vi "Desktop Main.vi"() -> ()   [LabVIEW 2016]
doc: "This VI implements the framework and scheduler for your robotics program. It should not be necessary to modify the framework. You are expected to add your code to the VIs called from Robot Main - the ones located in the Team Code folder within the project."
uses:
  Vision Server/Vision Server.lvclass
panel:
  in  "ADB Path":path caption="ADB path (if not in Windows PATH)"
  out "Distance":dbl
  in  "Goal Height":dbl
  out "Angle":dbl
  out "Connected?":bool
  out "Targets Detected:":i32
  out "Coords":cluster{"X":dbl, "Y":dbl}[](graph) caption="Frist Target Coordinates"
  out "Time Delay":u32(graph)
  in  "stop":bool
  in  "error in":errorcluster
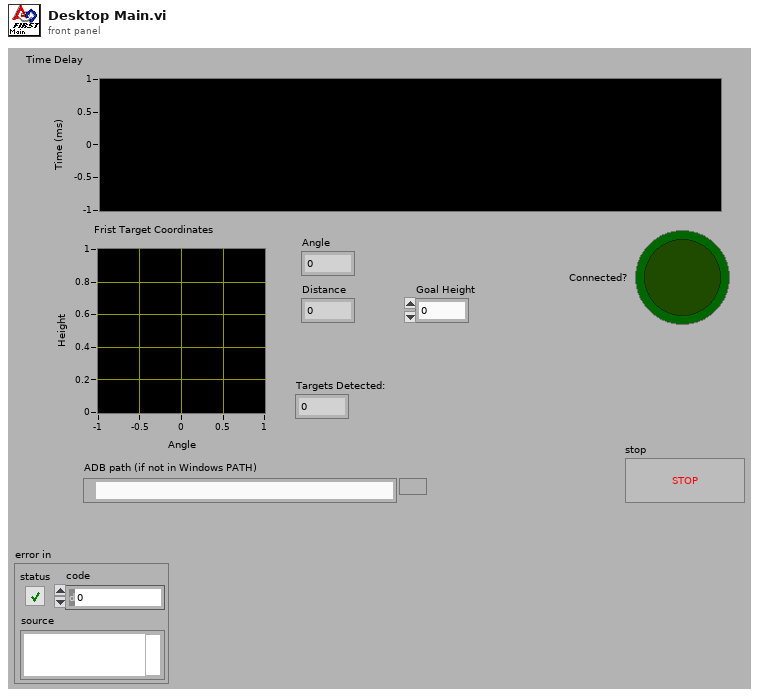
[diagram p1: front panel]
types:
  T1 = typedef "Vision Server.lvclass/Vision Server Ref.ctl" = cluster{"DVR":refnum<data-value>}
  T2 = typedef "Vision Server.lvclass/Target Listener Queue.ctl" = refnum<queue>
  T3 = typedef "Vision Server.lvclass/Target Vector.ctl" = cluster{"y":dbl, "z":dbl}
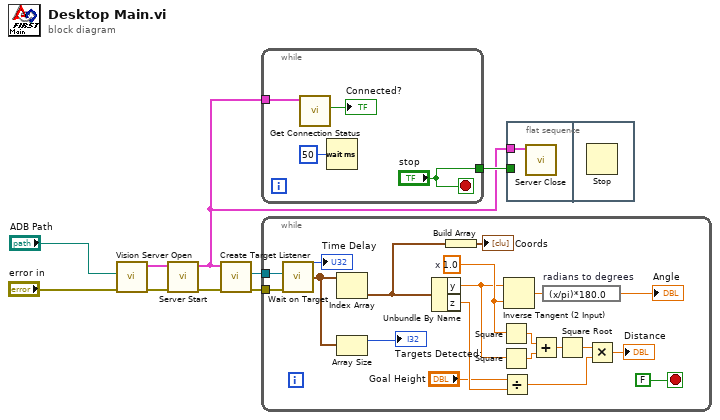
[diagram p0: block diagram]
diagram:
  n1 = call "Vision Server Open.vi"("error in (no error)"="error in", "ADB Path (Optional)"="ADB Path") -> ("error out"=w6:errorcluster, "VisionServerRef out"=w4:T1)  [unwired: 8 in]
  n2 = call "Server Start.vi"("error in"=w6, "VisionServerRef in"=w4) -> ("error out"=w5:errorcluster, "VisionServerRef out"=w2:T1)  [unwired: 8 in]
  n3 = call "Create Target Listener.vi"("error in"=w5, "VisionServerRef in"=w2) -> ("error out"=w9:errorcluster, "queue out"=w3:T2)  [unwired: 7 in, 1 out]
  n4 = while {
    tunnel: ["stop"] -> w8
    tunnel: w2 -> [w11]
    stop <- "stop" stop-if-true
    n5 = call "Get Connection Status.vi"("VisionServerRef in"=w11) -> ("connected?"=→"Connected?":bool)  [unwired: 8 in, 2 out]
    n6 = Wait (ms)(milliseconds to wait=u32 50) -> ()  [unwired: 1 out]
  }
  n7 = while {
    tunnel: w9 -> [w33]
    tunnel: w3 -> [w14]
    stop <- FALSE stop-if-true
    w24 = 1.0  # x
    n8 = call "Wait on Target.vi"("error in (no error)"=w33, "queue in"=w14) -> ("targets"=w30:T3[], "timestamp"=→"Time Delay":u32)  [unwired: 6 in, 2 out]
    n9 = Index Array(array=w30) -> (element=w27:T3)  [unwired: 1 in]
    n10 = Array Size(array=w30) -> (size(s)=→"Targets Detected:":i32)
    n11 = Unbundle By Name(w27) -> ("y"=w20:dbl, "z"=w18:dbl)
    n12 = Build Array(w27) -> (→"Coords":T3[])
    n13 = Square(x=w24) -> (x^2=w23:dbl)
    n14 = Square(x=w20) -> (x^2=w22:dbl)
    n15 = Divide(x="Goal Height", y=w18) -> (x/y=w16:dbl)
    n16 = Inverse Tangent (2 Input)(1:w24, 2:w20) -> (0:w26:dbl)
    n17 = Add(x=w23, y=w22) -> (x+y=w21:dbl)
    n18 = expression code="(x/pi)*180.0" "radians to degrees"(w26) -> (→"Angle":dbl)
    n19 = Square Root(x=w21) -> (sqrt(x)=w19:dbl)
    n20 = Multiply(x=w19, y=w16) -> (x*y=→"Distance":dbl)
  }
  n21 = flat-sequence {
    tunnel: w8 -> [_]
    tunnel: w2 -> [w34]
    frame #0 {
      n22 = call "Server Close.vi"("VisionServerRef in"=w34) -> ()  [unwired: 9 in, 2 out]
    }
    frame #1 {
      n23 = Stop() -> ()  [unwired: 1 in]
    }
  }
